vi "Get All Selected Objects.vi"() -> ()   [LabVIEW 2019]
doc: "Demonstrates the use of the Selection List[] property in VI Scripting to read the current selection on the front panel or block diagram."
panel:
  out "Currently Selected Objects":string[](array[string])
  # "Overview: Demonstrates the use of the Selection List[] property in VI Scripting to read the current selection on the front panel or block diagram.\nInstructions:\n1. Open Test - Selection List Target.vi.\n2. Select one or more objects on the front panel or block diagram.\n3. Run this VI. Whatever selection you previously made will be reflected in the Currently Selected Objects list below."
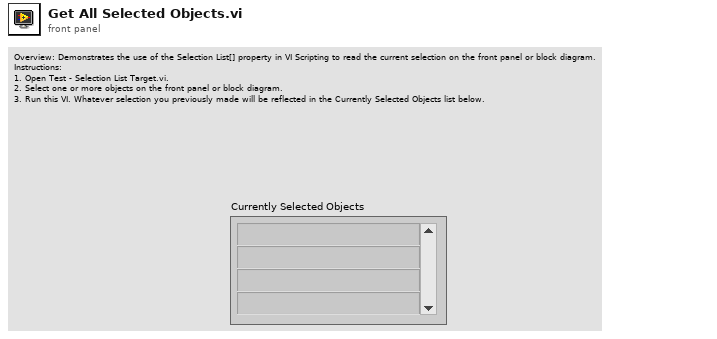
[diagram p1: front panel]
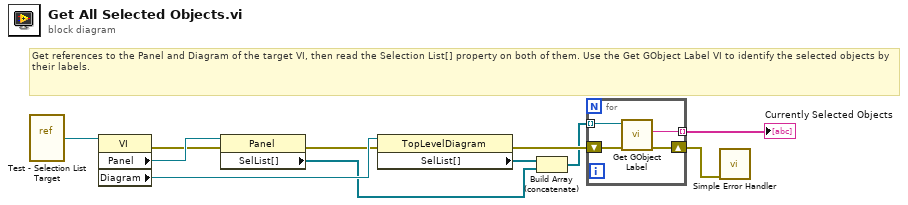
[diagram p0: block diagram]
diagram:
  # "Get references to the Panel and Diagram of the target VI, then read the Selection List[] property on both of them. Use the Get GObject Label VI to identify the selected objects by their labels."
  n1 = vi-ref "Test - Selection List Target.vi"() -> (w11:refnum<vi>)
  n2 = property class="VI"(reference=w11) -> (error out=w6:errorcluster, "Panel"=w9:refnum<vi>, "Diagram"=w8:refnum<vi>)  [unwired: 1 in, 1 out]
  n3 = property class="Panel"(reference=w9, error in=w6) -> (error out=w5:errorcluster, "SelList[]"=w2:refnum<vi>[])  [unwired: 1 out]
  n4 = property class="TopLevelDiagram"(reference=w8, error in=w5) -> (error out=w4:errorcluster, "SelList[]"=w7:refnum<vi>[])  [unwired: 1 out]
  n5 = Build Array (concatenate)(w7, w2) -> (w1:refnum<vi>[])
  n6 = for {
    tunnel: [w14] -> w10 mode=indexing
    tunnel: w1 -> [w15] mode=indexing
    shift-right: [w12] -> w3
    shift-left: w4 -> [w13]
    n7 = call <vilib>:"Get GObject Label.vi"("error in (no error)"=w13, "GObject"=w15) -> ("error out"=w12:errorcluster, "Object Label"=w14:string)  [unwired: 5 in, 3 out]
  }
  "Currently Selected Objects" <- w10
  n8 = call <vilib>:"Simple Error Handler.vi"("error in (no error)"=w3) -> ()  [unwired: 4 in, 5 out]
